vi "QTab DEMO-Sub3.vi"() -> ()   [LabVIEW 2020]
panel:
  in  "String":string="5555"
  in  "Boolean":bool
  out "Gauge":dbl(knob) scale=0.0..10.0
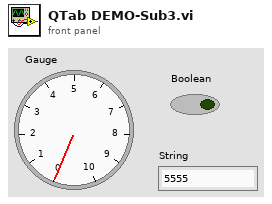
[diagram p1: front panel]
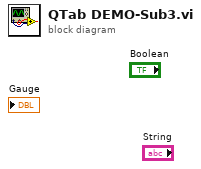
[diagram p0: block diagram]
diagram:
